vi "MBUS_BuildMbusData.vi"(8 "data":u16[](array[numeric]), 9 "NumRegs":u16, 10 "StartingAddr":u16, 11 "MFC":u8) -> (2 "sizeOfReturnData":u16, 3 "dataOut":string)   [LabVIEW 2012, in "MBUS_Modbus.lvlib"]
uses:
  MBUS_Modbus.lvlib
panel:
  out "Array":u8[](array[numeric])
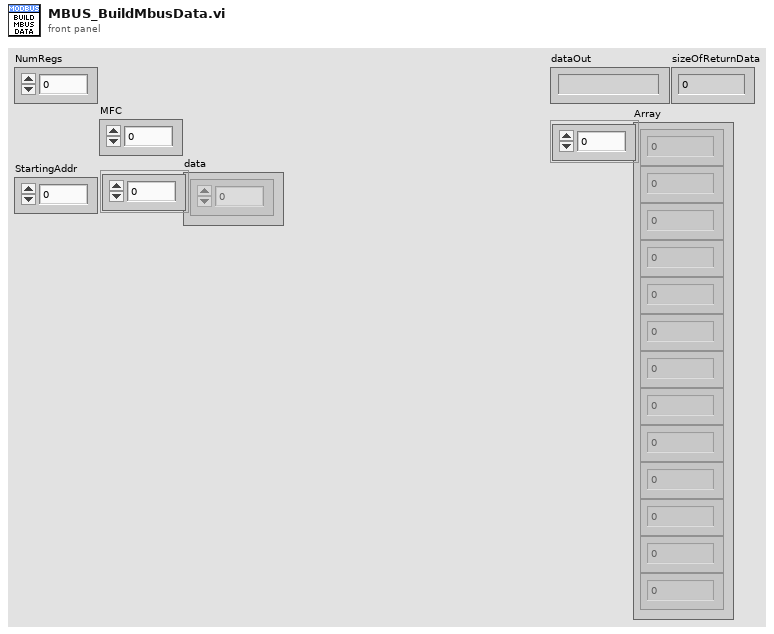
[diagram p1: front panel]
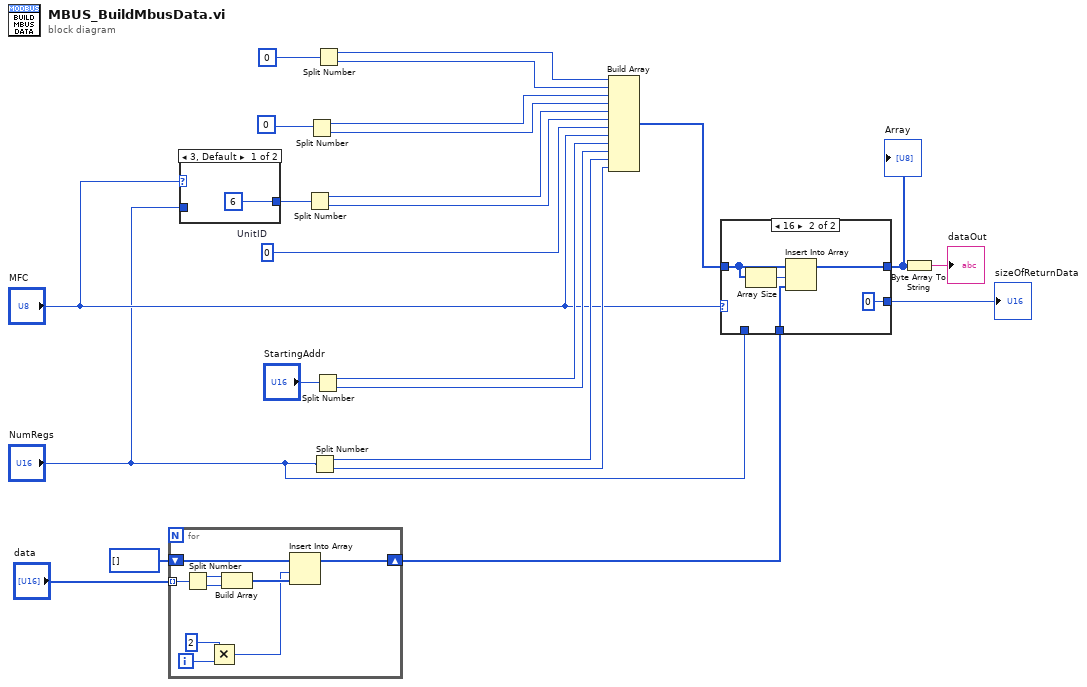
[diagram p0: block diagram]
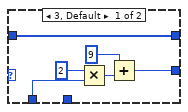
[diagram p2: hidden frame]
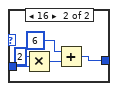
[diagram p3: hidden frame]
diagram:
  w18 = u8 0  # UnitID
  n1 = for {
    tunnel: "data" -> [w33] mode=indexing
    shift-right: [w26] -> w4
    shift-left: u8[] [] -> [w25]
    i -> [w29]
    n2 = Split Number(x=w33) -> (hi(x)=w32:u8, lo(x)=w31:u8)
    n3 = Multiply(x=2, y=w29) -> (x*y=w27:i32)
    n4 = Build Array(w32, w31) -> (w30:u8[])
    n5 = Insert Into Array(array=w25, index=w27, new element=w30) -> (w26:u8[])
  }
  n6 = case shown="3, Default" "MFC" {
    tunnel: [u16 6 ("x") w36] -> w12
    tunnel: "NumRegs" -> [_ w39]
    frame 3, Default {
    }
    frame 16 {
      n7 = Multiply(x=u16 2, y=w39) -> (x*y=w37:u16)
      n8 = Add(x=u16 6, y=w37) -> (x+y=w36:u16)
    }
  }
  n9 = Split Number(x=w12) -> (hi(x)=w20:u8, lo(x)=w19:u8)
  n10 = Split Number(x=u16 0) -> (hi(x)=w22:u8, lo(x)=w21:u8)
  n11 = Split Number(x="NumRegs") -> (hi(x)=w11:u8, lo(x)=w10:u8)
  n12 = Split Number(x="StartingAddr") -> (hi(x)=w16:u8, lo(x)=w15:u8)
  n13 = Split Number(x=u16 0) -> (hi(x)=w24:u8, lo(x)=w23:u8)
  n14 = Build Array(w24, w23, w22, w21, w20, w19, w18, "MFC", w16, w15, w11, w10) -> (w8:u8[])
  n15 = case shown="16" "MFC" {
    tunnel: w8 -> [w45 w48]
    tunnel: [w45 w50] -> w7
    tunnel: w4 -> [_ w47]
    tunnel: "NumRegs" -> [w44 _]
    tunnel: [w40 u16 0] -> w1
    frame 3, Default {
      n16 = Multiply(x=u16 2, y=w44) -> (x*y=w42:u16)
      n17 = Add(x=u16 9, y=w42) -> (x+y=w40:u16)
    }
    frame 16 {
      n18 = Array Size(array=w48) -> (size(s)=w49:i32)
      n19 = Insert Into Array(array=w48, index=w49, new element=w47) -> (w50:u8[])
    }
  }
  "Array" <- w7
  "sizeOfReturnData" <- w1
  n20 = Byte Array To String(unsigned byte array=w7) -> (string=→"dataOut":string)
